vi "Dashboard Main.vi"() -> ()   [LabVIEW 2015]
uses:
  <vilib>/Utility/miscctls.llb/LVRowAndColumnTypeDef.ctl
  <vilib>/event_ctls.llb/eventvkey.ctl
  <vilib>/Rock Robotics/WPI/Dashboard/WPI_DashboardLogging Global.vi
  <vilib>/Rock Robotics/Network Tables/NT Read Numeric Array.vi
  <vilib>/Rock Robotics/Network Tables/NT Read Boolean.vi
  <vilib>/Utility/config.llb/Write Key (String).vi
  <vilib>/Utility/config.llb/Write Key (I32).vi
  <vilib>/Utility/config.llb/NI_LVConfig.lvlib
panel:
  in  "TCP":refnum<k5>
  in  "Rec Mode":enum32{"Stop", "Record", "Playback"}(radio)
  in  "Vision":u16(ring) items=["Camera Off", "USB Camera SW", "USB Camera HW", "IP Camera"]
  out "Camera IP":string
  out "Image Message":string="Timeout in Camera Communications"
  in  "Dashboard Tab":T1(tab)
  in  "Select Auto":string(combo)
  out "NT Connection":bool
  in  "Camera Settings":T2={"Frame Rate"=30, "Compression"=30, "Size"=1} {"Frame Rate" scale=1.0..30.0; "Size" items=["640x480", "320x240", "160x120"]}
  out "MotorChart R":cluster{"Numeric":dbl, "Numeric":dbl}(graph)
  out "MotorChart L":T3(graph)
  out "MotorSliders R":cluster{"MotorSlide1":dbl, "MotorSlide2":dbl} {"MotorSlide2" scale=-1.0..1.0 scale format="%#_2e"; "MotorSlide1" scale=-1.0..1.0 scale format="%#_2e"}
  out "MotorSliders L":T4 {"MotorSlide4 2" scale=0.0..14.0 scale format="%#_2e"; "MotorSlide2" scale=-1.0..1.0 scale format="%#_2e"; "MotorSlide1" scale=-1.0..1.0 scale format="%#_2e"}
  out "Gyro":dbl(knob) scale=0.0..360.0
  out "JS1 Z":dbl(slide) scale=-1.0..1.0 scale format="%#_2e"
  out "JS1 Graph":cluster{"X":dbl, "Y":dbl}[](graph)
  out "JS1 Buttons":T5
  out "JS2 Z":dbl(slide) scale=-1.0..1.0 scale format="%#_2e"
  out "JS2 Graph":cluster{"X":dbl, "Y":dbl}[](graph)
  out "JS2 Buttons":T5
  out "Mode":T6(ring)=enum."Auto Disabled"
  in  "DB Camera Config":bool
  out "fps":dbl format="%#.1g"
  out "Mbps":dbl format="%#.1g"
  out "Mbps LED":bool
  in  "DB/String 9":string
  in  "DB/String 8":string
  in  "DB/String 7":string
  in  "DB/String 6":string
  in  "DB/String 5":string
  in  "DB/String 4":string
  in  "DB/String 3":string
  in  "DB/String 2":string
  in  "DB/String 1":string
  in  "DB/String 0":string
  in  "DB/Slider 0":dbl(slide) scale=0.0..5.0
  in  "DB/Slider 1":dbl(slide) scale=0.0..5.0
  in  "DB/Slider 2":dbl(slide) scale=0.0..5.0
  in  "DB/Slider 3":dbl(slide) scale=0.0..5.0
  out "DB/LED 3":bool
  out "DB/LED 2":bool
  out "DB/LED 1":bool
  out "DB/LED 0":bool
  in  "DB/Button 3":bool
  in  "DB/Button 2":bool
  in  "DB/Button 1":bool
  in  "DB/Button 0":bool caption="New Name"
  in  "Position":enum16{"No Launch", "3"}(ring)
  in  "Defense":T7(ring)
  out "Air Pressure":dbl
  out "Ball In Catapult":bool
  out "Climbing Only":bool
  in  "Test Slider":dbl(slide) scale=0.0..100.0 scale format="%#_3g"
  in  "On/Off":bool caption="Solenoid"
  in  "Test Name":u16(ring) items=["Select the test to run..."]
  in  "Test Tree":string(tree)
  in  "Motor":cluster{"Value":dbl, "Enable":bool} {"Value" scale=-1.0..1.0 scale format="%#_3g"}
  out "Progress":T8 {"Test Progress" scale=0.0..100.0}
  in  "Rev/Fwd":cluster{"Forward":bool, "Reverse":bool}
  in  "Test Ring":u16(ring) items=["Monochrome", "Color"]
  out "Cmd Status":string
  in  "Execute Command":bool
  in  "Command Params":string[][](table)
  in  "Command Selection":i32(listbox)
  in  "CheckList":i32(listbox)
  out "Tree":string(tree)
  out "Camera Image":T9(plugin-control)
  out "Background":bool
  # "Left"
  # "Front"
  # "Right"
  # "Battery"
  # "Autonomus"
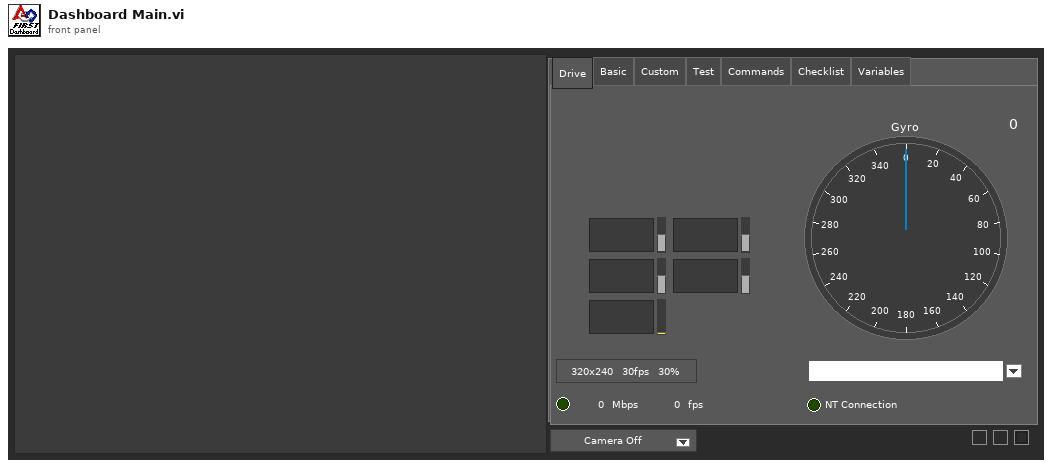
[diagram p1: front panel]
types:
  T1 = enum32{"Drive", "Basic", "Custom", "Test", "Commands", "Checklist", "Variables"}
  T2 = cluster{"Frame Rate":i32, "Compression":i32, "Size":u16}
  T3 = cluster{"Numeric":dbl, "Numeric":dbl, "Battery V":dbl}
  T4 = cluster{"MotorSlide1":dbl, "MotorSlide2":dbl, "MotorSlide4 2":dbl}
  T5 = cluster{bool, bool, bool, bool, bool, bool, bool, bool, bool, bool, bool, bool}
  T6 = enum8{"Tele-Op Disabled", "Tele-Op Enabled", "Auto Disabled", "Auto Enabled", "Test Disabled", "Test Enabled", "Disconnected", "No Code", "E-Stop"}
  T7 = enum16{"Rock Wall/Rough Terrain/Moat", "Ramp Parts", "Low Bar"}
  T8 = cluster{"Test Progress":u8, "Test Progress Text":string}
  T9 = typedef "IMAQ Image.ctl" = refnum<image>
  T10 = cluster{"IDs":cluster{"RPC field ID":u16, "Unique ID":u16}, "String":string}
  T11 = enum32{"Drive", "Basic", "Custom", "Test", "Checklist", "Variables"}
  T12 = typedef "Image Type" = u32
  T13 = cluster{"Camera Image":refnum<vi>, "Dashboard Tab":refnum<vi>, "Background":refnum<vi>, "Vision":refnum<vi>, "Rec Mode":refnum<vi>, "Test Slider":refnum<vi>, "On/Off ":refnum<vi>, "Test Ring":refnum<vi>, "Rev/Fwd":refnum<vi>, "Test Name":refnum<vi>, "Motor":refnum<vi>, "Progress":refnum<vi>, "CheckList":refnum<vi>, "Tree":refnum<vi>, "Test Tree":refnum<vi>, "Command Params":refnum<vi>, "Command Selection":refnum<vi>, "Execute Command":refnum<vi>, "Cmd Status":refnum<vi>}
  T14 = cluster{"Error Strings":string, "Disable Counts":cluster{u16, u16}, "Rail Faults":cluster{u16, u16, u16}, "Robot IP":string, "DB Mode":u8, "Event Info":cluster{"Name":string, "Type":u8, "Number":u16, "Replay":u8}, "Camera Addr":string}
  T15 = cluster{"Storage":cluster{"Disk Free":u64, "RAM Block":u32, "RAM free":u32}, "CPU Utilization":cluster{"CPU % ISR":sgl, "CPU % Time Crit":sgl, "CPU % Timed Str":sgl, "CPU % High":sgl, "CPU % Above":sgl, "CPU % Normal":sgl, "CPU % Low":sgl}, "CAN":cluster{"% Bus Utilization":sgl, "Bus Off Cnt":u32, "TX_FIFO Full Cnt":u32, "Receive Error Cnt":u8, "Transmit Error Cnt":u8}, "HID":cluster{"HID Outputs":u32, "Rumble Low":u16, "Rumble High":u16}[]}
  T16 = cluster{"Status bits":cluster{"Test Mode":bool, "Autonomous":bool, "Enabled":bool, "Code Start":bool, "Brownout":bool, "Reserved 2":bool, "Reserved 3":bool, "E-Stop":bool}, "Code Trace":cluster{"Disabled":bool, "TeleOp":bool, "Auto":bool, "Test":bool}, "Controller Type":enum16{"unknown", "cRIO", "roboRio"}, "Code?":enum16{"unknown", "noCode", "code"}, "Battery V":dbl}
  T17 = cluster{"Control Bits":cluster{"TestMode":bool, "Autonomous":bool, "Enabled":bool, "FMS Present":bool, bool, bool, bool, "E-Stop":bool}, "Team Station ":u8, "Countdown":sgl, "Joystick Values":cluster{"Axes":dbl[], "Buttons":bool[], "POVs":i16[]}[]}
  T18 = cluster{"Axes":dbl[], "Buttons":bool[], "POVs":i16[]}[]
  T19 = cluster{"Axes":dbl[], "Buttons":bool[], "POVs":i16[]}
  T20 = cluster{"Buttons[0]":bool, "Buttons[1]":bool, "Buttons[2]":bool, "Buttons[3]":bool, "Buttons[4]":bool, "Buttons[5]":bool, "Buttons[6]":bool, "Buttons[7]":bool, "Buttons[8]":bool, "Buttons[9]":bool, "Buttons[10]":bool, "Buttons[11]":bool}
  T21 = typedef "NI_LVConfig.lvlib/Config Data RefNum.ctl" = refnum<k1>
  T22 = cluster{"Operation":enum16{"Update", "Clear"}, "Color Box":u32}[]
  T23 = typedef "eventvkey.ctl" = enum16{"ASCII", "Enter", "Return", "Shift", "Ctrl", "Alt", "Cmd", "Opt", "Caps", "NumLock", "Clear", "Break", "Up", "Down", "Left", "Right", "Insert", "Delete", "Home", "End", "PageUp", "PageDown", "Escape", "Help", "Pause", "ScrollLock", "F1", "F2", "F3", "F4", "F5", "F6", "F7", "F8", "F9", "F10", "F11", "F12", "F13", "F14", "F15", "F16", "F17", "F18", "F19", "F20", "F21", "F22", "F23", "F24", "Play", "VolumeUp", "VolumeDown", "Mute", "Two Byte Char"}
  T24 = cluster{"Image Size":bool, "Image Type":bool, "Pixel Value":bool, "ROI Information":bool, "Zoom Factor":bool}
  T25 = enum8{"Enabled", "Disabled", "Disabled and Grayed Out"}
  T26 = cluster{"Operation":enum16{"Update", "Clear"}, "Color Box":u32}
  T27 = typedef "LVRowAndColumnTypeDef.ctl" = cluster{"Row":i32, "Column":i32}
  T28 = cluster{"Shift":bool, "Ctrl":bool, "Alt":bool, "Cmd":bool, "Opt":bool}
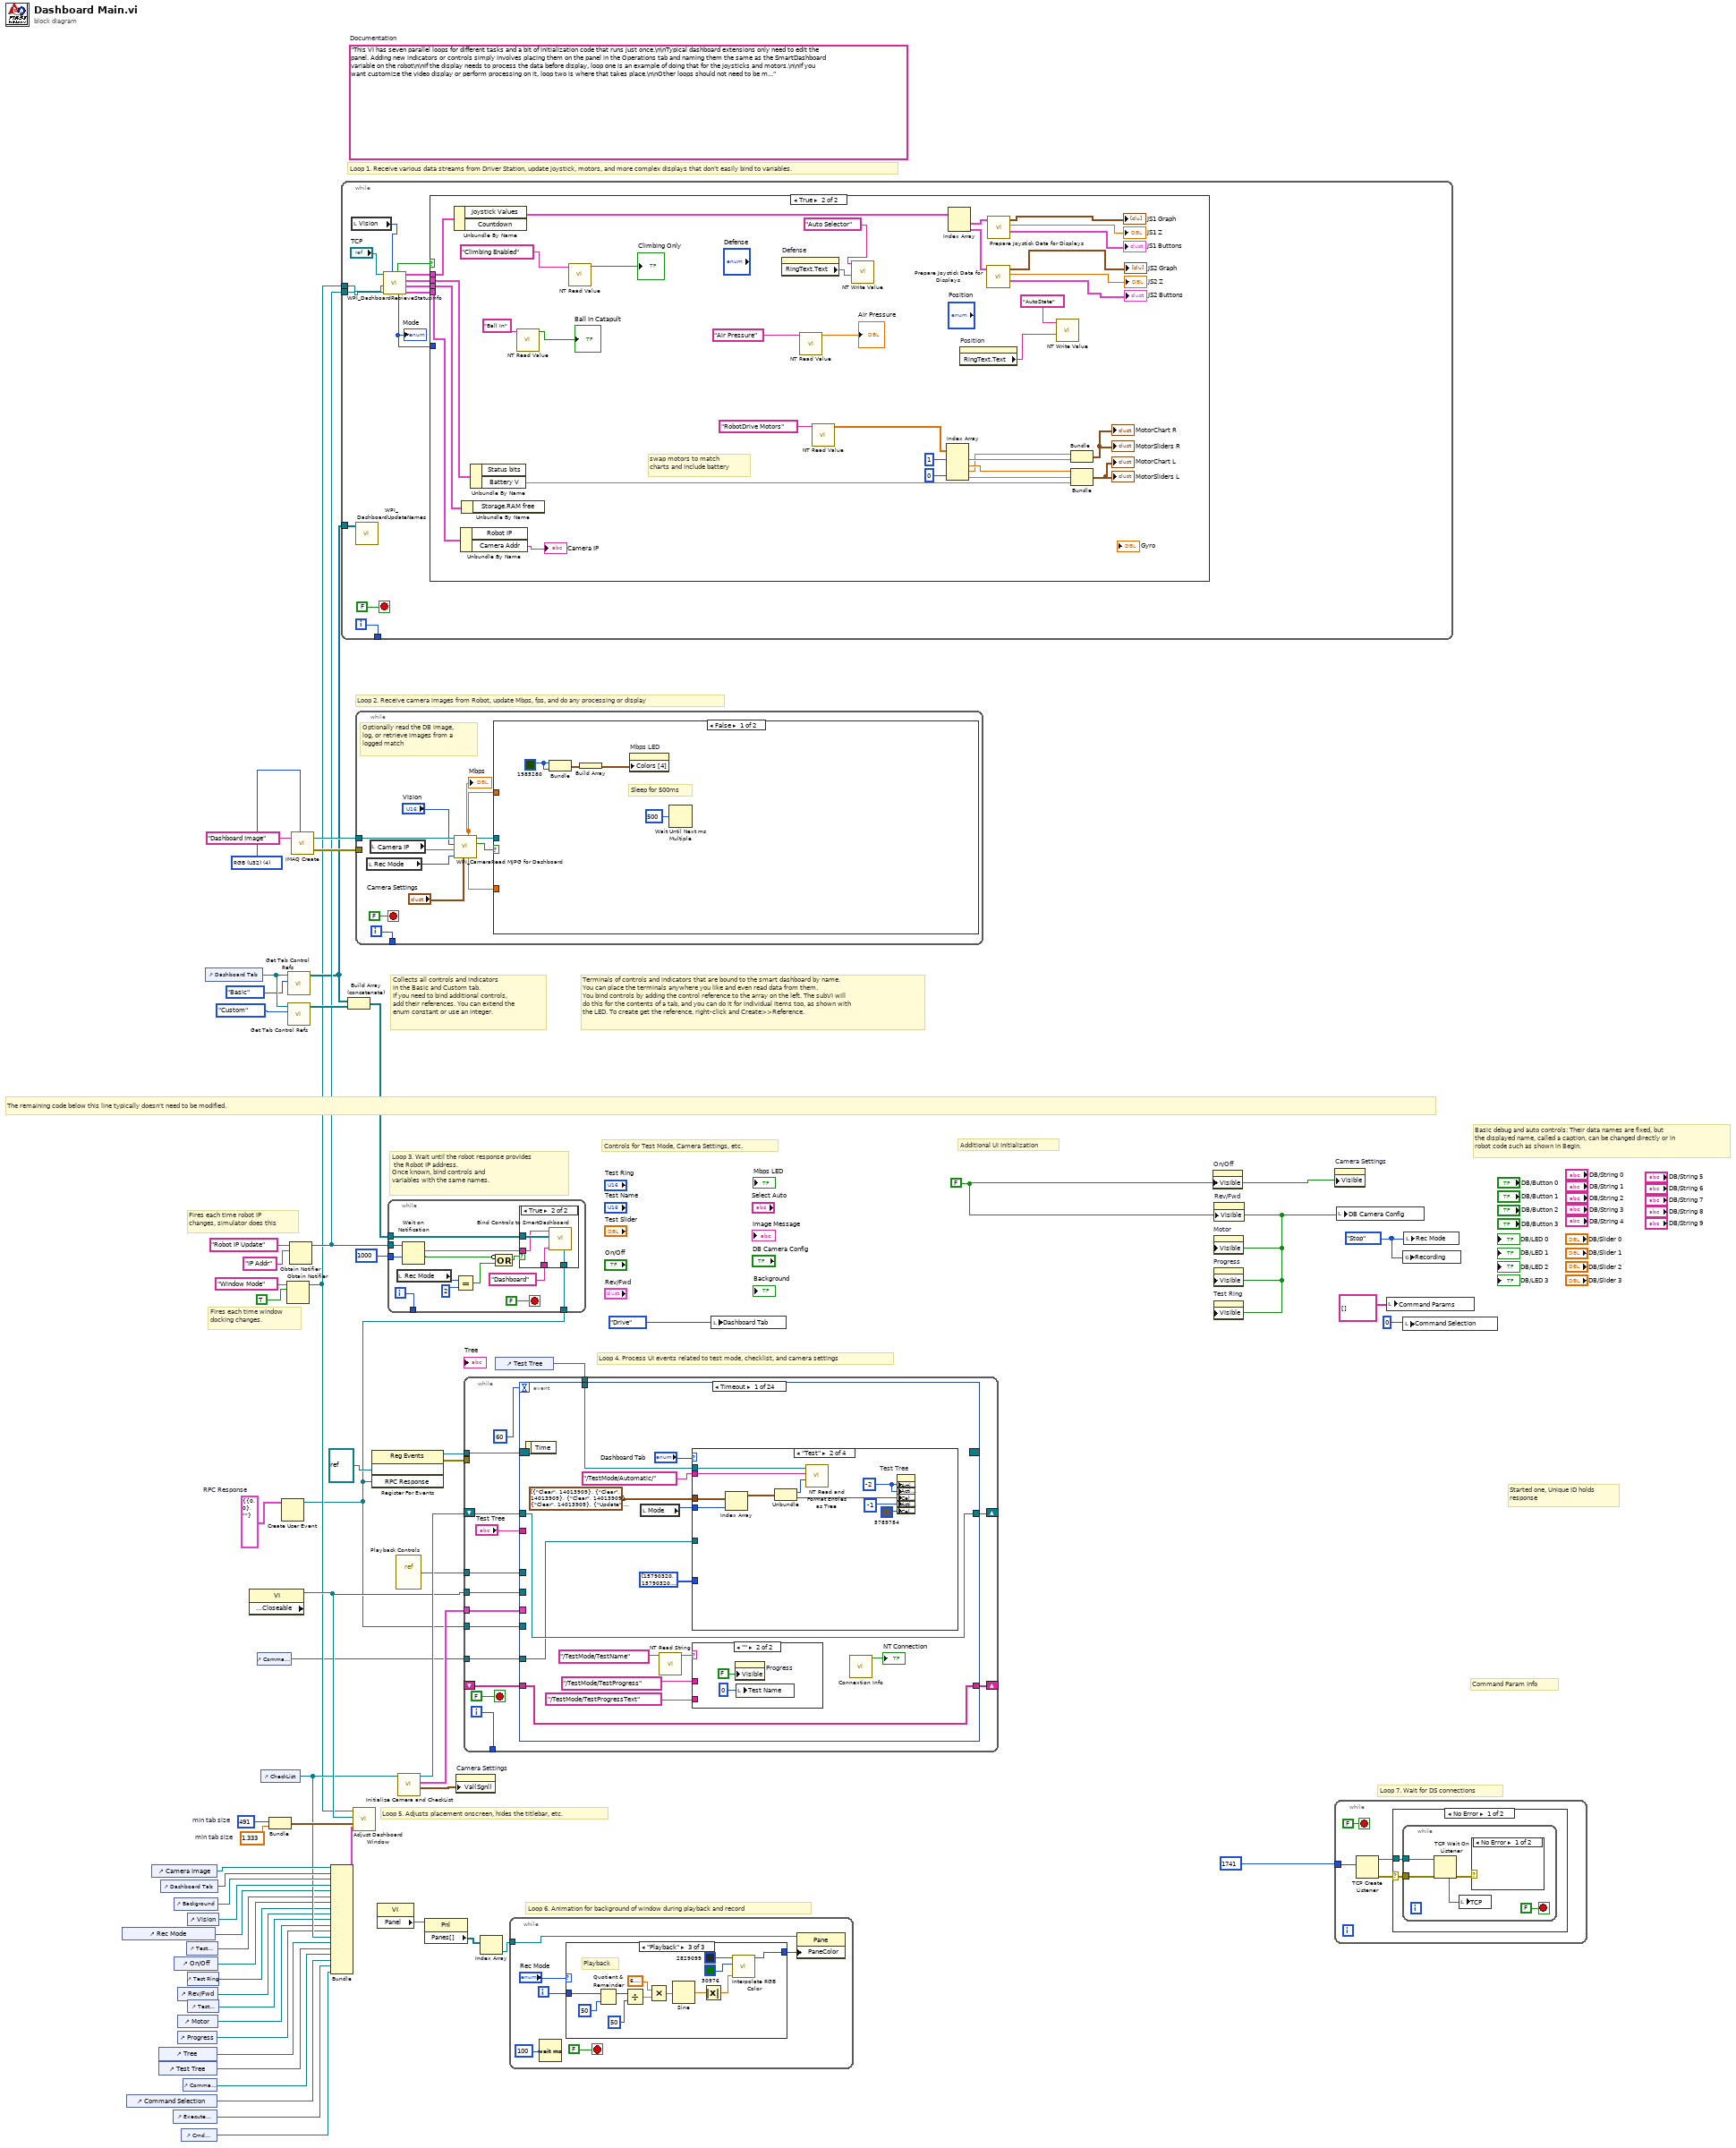
[diagram p0: block diagram]
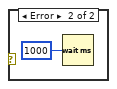
[diagram p2: hidden frame]
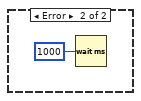
[diagram p3: hidden frame]
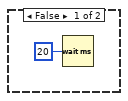
[diagram p4: hidden frame]
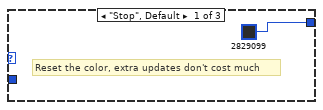
[diagram p5: hidden frame]
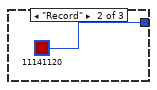
[diagram p6: hidden frame]
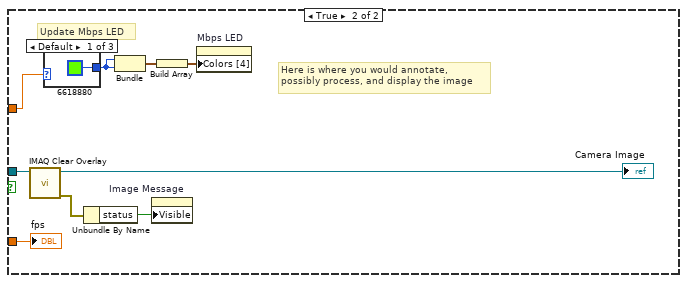
[diagram p8: hidden frame]
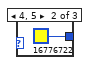
[diagram p9: hidden frame]
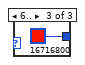
[diagram p10: hidden frame]
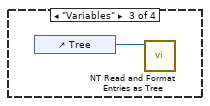
[diagram p12: hidden frame]
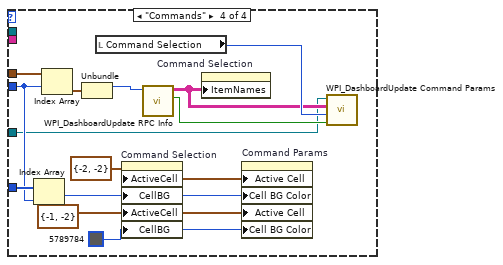
[diagram p13: hidden frame]
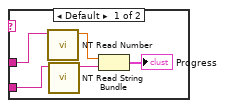
[diagram p14: hidden frame]
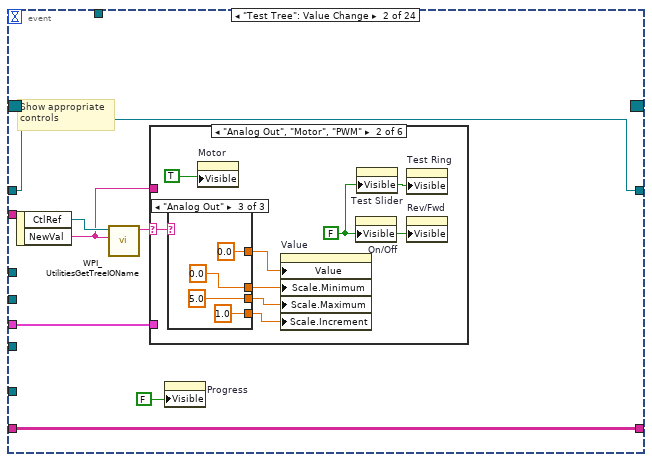
[diagram p15: hidden frame]
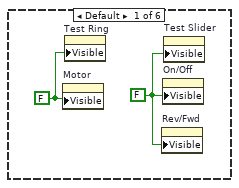
[diagram p16: hidden frame]
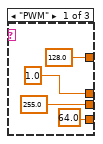
[diagram p17: hidden frame]
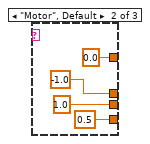
[diagram p18: hidden frame]
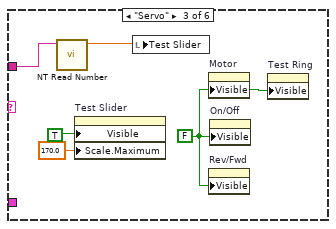
[diagram p19: hidden frame]
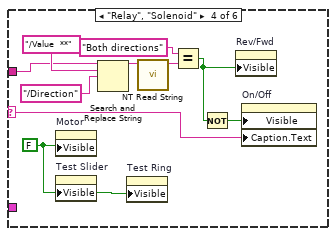
[diagram p20: hidden frame]
diagram:
  w7 = T10 {"IDs"={"RPC field ID"=0, "Unique ID"=0}, "String"=""}  # RPC Response
  w33 = 491  # min tab size
  w32 = 1.333  # min tab size
  w41 = enum32{"Stop", "Record", "Playback"}."Stop" ("Rec Mode")
  w15 = FALSE ("Visible")
  (unwired) "This VI has seven parallel loops for different tasks and a bit of initialization code that runs just once.\n\nTypical dashboard extensions only need to edit the panel. Adding new indicators or controls simply involves placing them on the panel in the Operations tab and naming them the same as the SmartDashboard variable on the robot\n\nIf the display needs to process the data before display, loop one is an example of doing that for the joysticks and motors.\n\nIf you want customize the video display or perform processing on it, loop two is where that takes place.\n\nOther loops should not need to be modified. They are pretty standard, and document the task they perform."  # Documentation
  w61 = T12 4 items=["Grayscale (U8)", "Grayscale (I16)", "Grayscale (SGL)", "Complex (CSG)", "RGB (U32)", "HSL (U32)", "RGB (U64)"] ("Image Type")
  # "Command Param Info"
  # "Started one, Unique ID holds\nresponse"
  # "Loop 7. Wait for DS connections"
  # "Basic debug and auto controls: Their data names are fixed, but\nthe displayed name, called a caption, can be changed directly or in\nrobot code such as shown in Begin."
  # "Controls for Test Mode, Camera Settings, etc."
  # "Additional UI Initialization"
  # "Loop 6. Animation for background of window during playback and record"
  # "Fires each time robot IP\nchanges, simulator does this"
  # "Fires each time window\ndocking changes."
  # "Collects all controls and indicators\nin the Basic and Custom tab.\nIf you need to bind additional controls,\nadd their references. You can extend the\nenum constant or use an integer."
  # "The remaining code below this line typically doesn't need to be modified."
  # "Loop 4. Process UI events related to test mode, checklist, and camera settings"
  # "Terminals of controls and indicators that are bound to the smart dashboard by name.\nYou can place the terminals anywhere you like and even read data from them.\nYou bind controls by adding the control reference to the array on the left. The subVI will\ndo this for the contents of a tab, and you can do it for individual items too, as shown with\nthe LED. To create get the reference, right-click and Create>>Reference."
  # "Loop 3. Wait until the robot response provides\n the Robot IP address.\nOnce known, bind controls and\nvariables with the same names."
  # "Loop 5. Adjusts placement onscreen, hides the titlebar, etc."
  # "Loop 1. Receive various data streams from Driver Station, update joystick, motors, and more complex displays that don't easily bind to variables."
  # "Loop 2. Receive camera images from Robot, update Mbps, fps, and do any processing or display"
  n1 = control-ref of="Rec Mode"() -> (w21:refnum<vi>)
  n2 = control-ref of="Command Selection"() -> (w6:refnum<vi>)
  n3 = control-ref of="Camera Image"() -> (w36:refnum<vi>)
  n4 = control-ref of="Tree"() -> (w25:refnum<vi>)
  n5 = control-ref of="Test Tree"() -> (w24:refnum<vi>)
  n6 = control-ref of="Dashboard Tab"() -> (w35:refnum<vi>)
  n7 = control-ref of="Execute Command"() -> (w8:refnum<vi>)
  n8 = control-ref of="Background"() -> (w30:refnum<vi>)
  n9 = control-ref of="On/Off"() -> (w19:refnum<vi>)
  n10 = control-ref of="Progress"() -> (w16:refnum<vi>)
  n11 = control-ref of="Rev/Fwd"() -> (w17:refnum<vi>)
  n12 = control-ref of="Motor"() -> (w22:refnum<vi>)
  n13 = control-ref of="Cmd Status"() -> (w2:refnum<vi>)
  n14 = control-ref of="Command Params"() -> (w9:refnum<vi>)
  n15 = control-ref of="Test Slider"() -> (w20:refnum<vi>)
  n16 = control-ref of="Vision"() -> (w34:refnum<vi>)
  n17 = control-ref of="Test Ring"() -> (w18:refnum<vi>)
  n18 = control-ref of="Test Name"() -> (w23:refnum<vi>)
  n19 = control-ref of="Dashboard Tab"() -> (w39:refnum<vi>)
  n20 = property class="VI" props=["Front Panel.Closeable"]() -> (reference out=w40:refnum<vi>)  [unwired: 2 in, 2 out]
  n21 = control-ref of="Command Params"() -> (w1:refnum<vi>)
  n22 = control-ref of="CheckList"() -> (w26:refnum<vi>)
  n23 = Bundle("min tab size"=w33, "min tab size"=w32) -> (w31:cluster{"min tab size":i32, "min tab size":dbl})  [unwired: 1 in]
  n24 = Create User Event(user event datatype=w7) -> (user event=w3:refnum<user-event>)  [unwired: 1 in, 1 out]
  n25 = Obtain Notifier(name (unnamed)="Window Mode", notification data type=TRUE) -> (notifier out=w12:refnum<notifier>)  [unwired: 2 in, 2 out]
  n26 = call <vilib>:"Get Tab Control Refs.vi"("Page Index"=T11."Basic" ("Dashboard Tab"), "TabControl in"=w39) -> ("ControlsOnPage"=w13:refnum<vi>[])  [unwired: 9 in]
  n27 = call <vilib>:"Get Tab Control Refs.vi"("Page Index"=T11."Custom" ("Dashboard Tab"), "TabControl in"=w39) -> ("ControlsOnPage"=w38:refnum<vi>[])  [unwired: 9 in]
  n28 = Obtain Notifier(name (unnamed)="Robot IP Update", notification data type="IP Addr" ("name (unnamed)")) -> (notifier out=w14:refnum<notifier>)  [unwired: 2 in, 2 out]
  n29 = call "IMAQ Create"("Image Name"="Dashboard Image", "Image Type"=w61) -> ("New Image"=w59:T9, "error out"=w58:errorcluster)  [unwired: 2 in, 1 out]
  n30 = Bundle("Camera Image"=w36, "Dashboard Tab"=w35, "Background"=w30, "Vision"=w34, "Rec Mode"=w21, "Test Slider"=w20, "On/Off"=w19, "Test Ring"=w18, "Rev/Fwd"=w17, "Test Name"=w23, "Motor"=w22, "Progress"=w16, "CheckList"=w26, "Tree"=w25, "Test Tree"=w24, "Command Params"=w9, "Command Selection"=w6, "Execute Command"=w8, "Cmd Status"=w2) -> (w27:T13)  [unwired: 1 in]
  n31 = while {
    tunnel: [w73] -> _
    tunnel: w14 -> [w67]
    tunnel: w13 -> [w66]
    tunnel: w12 -> [w62]
    i -> [w73]
    stop <- FALSE stop-if-true
    n32 = local read "Vision"() -> (w64:u16)
    n33 = call <vilib>:"WPI_DashboardUpdateNames.vi"("Controls on Tab"=w66) -> ()  [unwired: 11 in]
    n34 = call <vilib>:"WPI_DashboardRetrieveStatusInfo.vi"("Vision"=w64, "Binding Refnum"=w67, "Window Mode Notifier"=w62, "TCP Cnx"="TCP") -> ("Power and Errors"=w68:T14, "Robot Metrics"=w71:T15, "Status Info"=w72:T16, "Control Info"=w69:T17, "Robot Mode"=w65:T6, "Process?"=w70:bool)  [unwired: 2 in]
    "Mode" <- w65
    n35 = case shown="True" w70 {
      tunnel: w72 -> [_ w110]
      tunnel: w71 -> [_ w109]
      tunnel: w69 -> [_ w108]
      tunnel: w68 -> [_ w107]
      tunnel: w65 -> [_ _]
      frame False {
        n36 = Wait (ms)(milliseconds to wait=u32 20) -> ()  [unwired: 1 out]
      }
      frame True {
        # "swap motors to match\ncharts and include battery"
        n37 = Unbundle By Name(w108) -> ("Joystick Values"=w97:T18)  [unwired: 1 out]
        n38 = Unbundle By Name(w107) -> ("Camera Addr"=→"Camera IP":string)  [unwired: 1 out]
        n39 = Unbundle By Name(w109) -> ()  [unwired: 1 out]
        n40 = Unbundle By Name(w110) -> ("Battery V"=w98:dbl)  [unwired: 1 out]
        n41 = call-poly <vilib>:"NT Read Value.vi"("Name"="Ball In") -> ("Boolean"=→"Ball In Catapult":bool)  [unwired: 9 in, 1 out]
        n42 = call-poly <vilib>:"NT Read Value.vi"("Name"="Climbing Enabled") -> ("Boolean"=→"Climbing Only":bool)  [unwired: 9 in, 1 out]
        n43 = property on="Defense" class="Enum (strict)"() -> ("RingText.Text"=w78:string)  [unwired: 2 in, 2 out]
        n44 = call-poly <vilib>:"NT Read Value.vi"("Name"="Air Pressure") -> ("Numeric"=→"Air Pressure":dbl)  [unwired: 9 in, 1 out]
        n45 = call-poly <vilib>:"NT Read Value.vi"("Name"="RobotDrive Motors") -> ("Numeric Array"=w86:dbl[])  [unwired: 9 in, 1 out]
        n46 = call-poly <vilib>:"NT Write Value.vi"("String"=w78, "Name"="Auto Selector") -> ()  [unwired: 9 in, 1 out]
        n47 = Index Array(array=w86, index #1=1, index #4=0) -> (element #1=w102:dbl, element #2=w103:dbl, element #3=w101:dbl, element #4=w106:dbl)  [unwired: 2 in]
        n48 = Index Array(array=w97) -> (element #1=w96:T19, element #2=w91:T19)  [unwired: 2 in]
        n49 = property on="Position" class="Enum (strict)"() -> ("RingText.Text"=w77:string)  [unwired: 2 in, 2 out]
        n50 = call "Prepare Joystick Data for Displays.vi"("Joystick Values"=w91) -> ("Buttons"=→"JS2 Buttons":T20, "Z Axis"=→"JS2 Z":dbl, "Cartesian Data"=→"JS2 Graph":cluster{"X axis":dbl, "X axis":dbl}[])  [unwired: 8 in]
        n51 = call "Prepare Joystick Data for Displays.vi"("Joystick Values"=w96) -> ("Buttons"=→"JS1 Buttons":T20, "Z Axis"=→"JS1 Z":dbl, "Cartesian Data"=→"JS1 Graph":cluster{"X axis":dbl, "X axis":dbl}[])  [unwired: 8 in]
        n52 = call-poly <vilib>:"NT Write Value.vi"("String"=w77, "Name"="AutoState") -> ()  [unwired: 9 in, 1 out]
        n53 = Bundle("Numeric"=w101, "Numeric"=w102) -> (→"MotorChart R" →"MotorSliders R":cluster{"Numeric":dbl, "Numeric":dbl})  [unwired: 1 in]
        n54 = Bundle("Numeric"=w103, "Numeric"=w106, "Battery V"=w98) -> (→"MotorChart L" →"MotorSliders L":T3)  [unwired: 1 in]
      }
    }
  }
  n55 = Build Array (concatenate)(w13, w38) -> (w37:refnum<vi>[])
  n56 = call "Adjust Dashboard Window.vi"("Sizing Refnums"=w27, "Size Constraints"=w31, "VI"=w40, "WIn Mode"=w12) -> ()  [unwired: 8 in]
  n57 = while {
    tunnel: w59 -> [w119]
    tunnel: w58 -> [_]
    tunnel: [w120] -> _
    i -> [w120]
    stop <- FALSE stop-if-true
    # "Optionally read the DB image,\nlog, or retrieve images from a\nlogged match"
    n58 = local read "Rec Mode"() -> (w114:enum32{"Stop", "Record", "Playback"})
    n59 = local read "Camera IP"() -> (w112:string)
    n60 = call <vilib>:"WPI_CameraRead MJPG for Dashboard.vi"("Camera Settings"="Camera Settings", "Rec Mode"=w114, "Camera IP"=w112, "Camera Mode"="Vision", "Refnum in"=w119) -> ("Active"=w117:bool, "Refnum out"=w118:T9, "FPS"=w116:dbl, "Bandwidth (Mbps)"=w111:dbl)  [unwired: 3 in]
    "Mbps" <- w111
    n61 = case shown="False" w117 {
      tunnel: w118 -> [_ w129]
      tunnel: w111 -> [_ w128]
      tunnel: w116 -> [_ w126]
      frame False {
        w122 = u32 1985280 ("Color Box")
        # "Sleep for 500ms"
        n62 = Bundle("Color Box"=w122, "Color Box"=w122) -> (w124:cluster{"Color Box":u32, "Color Box":u32})  [unwired: 1 out]
        n63 = Build Array(w124) -> (w123:cluster{"Color Box":u32, "Color Box":u32}[])
        n64 = property on="Mbps LED" class="Bool (strict)"("Colors [4]"=w123) -> ()  [unwired: 2 in, 2 out]
        n65 = Wait Until Next ms Multiple(millisecond multiple=u32 500) -> ()  [unwired: 1 out]
      }
      frame True {
        # "Here is where you would annotate,\npossibly process, and display the image"
        # "Update Mbps LED"
        n66 = call "IMAQ Clear Overlay"("Image"=w129) -> ("error out"=w133:errorcluster, "Image Out"=→"Camera Image":T9)  [unwired: 2 in, 7 out]
        n67 = case shown="Default" w128 {
          tunnel: [u32 6618880 ("Color Box") u32 16776722 ("Color Box") u32 16716800 ("Color Box")] -> w130
          frame Default {
          }
          frame 4, 5 {
          }
          frame 6.. {
          }
        }
        n68 = Unbundle By Name(w133) -> ("status"=w134:bool)
        n69 = Bundle("Color Box"=w130, "Color Box"=w130) -> (w132:cluster{"Color Box":u32, "Color Box":u32})  [unwired: 1 out]
        n70 = property on="Image Message" class="Str"("Visible"=w134) -> ()  [unwired: 2 in, 2 out]
        n71 = Build Array(w132) -> (w131:cluster{"Color Box":u32, "Color Box":u32}[])
        n72 = property on="Mbps LED" class="Bool (strict)"("Colors [4]"=w131) -> ()  [unwired: 2 in, 2 out]
        "fps" <- w126
      }
    }
  }
  n73 = register-events(refnum<vi> refnum, w3) -> (reference out=w45:refnum<event-registration>, error out=w44:errorcluster)  [unwired: 2 in]
  n74 = property class="VI"() -> ("Panel"=w48:refnum<vi>)  [unwired: 2 in, 2 out]
  n75 = while {
    tunnel: w37 -> [w150]
    tunnel: w14 -> [w148]
    tunnel: [w146] -> _
    tunnel: u32 1000 ("milliseconds to wait") -> [w145]
    tunnel: w3 -> [w138]
    i -> [w146]
    stop <- FALSE stop-if-true
    n76 = local read "Rec Mode"() -> (w141:enum32{"Stop", "Record", "Playback"})
    n77 = Wait on Notification(notifier=w148, timeout in ms (-1)=w145) -> (notification=w147:string, timed out?=w143:bool)  [unwired: 2 in, 2 out]
    n78 = Equal?(x=w141, y=u16 2 ("Rec Mode")) -> (x = y?=w142:bool)
    n79 = Compound Arithmetic op=OR(invert w143, w142) -> (w144:bool)
    n80 = case shown="True" w144 {
      tunnel: w150 -> [_ w154]
      tunnel: w147 -> [_ w153]
      tunnel: "Dashboard" -> [_ w152]
      tunnel: w138 -> [_ w151]
      frame False {
      }
      frame True {
        n81 = call <vilib>:"Bind Controls to SmartDashboard.vi"("RPC ref"=w151, "Client Name"=w152, "Bound Control Refs"=w154, "Server IP Address"=w153) -> ()  [unwired: 8 in]
      }
    }
  }
  n82 = vi-ref "Playback Controls.vi"() -> (w46:refnum<vi>)
  n83 = call "Initialize Camera and CheckList.vi"("ListBox in"=w26) -> ("Cluster"=w52:cluster{"value":i32, "value":i32, "index":i32}, "Array"=w53:cluster{string[]}[], "File Refnum"=w51:T21)  [unwired: 8 in]
  n84 = property class="Pnl"(reference=w48) -> ("Panes[]"=w49:refnum<vi>[])  [unwired: 1 in, 2 out]
  n85 = property on="Camera Settings" class="Clust (strict)"("Val(Sgnl)"=w52) -> ()  [unwired: 2 in, 2 out]
  n86 = Index Array(array=w49) -> (element=w47:refnum<vi>)  [unwired: 1 in]
  n87 = control-ref of="Test Tree"() -> (w50:refnum<vi>)
  n88 = while {
    tunnel: w53 -> [w166]
    shift-right: [w165] -> _
    shift-left: w51 -> [w164]
    tunnel: [w163] -> _
    tunnel: w50 -> [w162]
    tunnel: w46 -> [w161]
    tunnel: w45 -> [w160]
    tunnel: w44 -> [_]
    tunnel: w40 -> [w159]
    tunnel: w3 -> [w158]
    tunnel: w1 -> [w157]
    shift-right: [w156] -> _
    shift-left: _ -> [w155]
    i -> [w163]
    stop <- FALSE stop-if-true
    n89 = event shown="[0] Timeout" {
      selector: w160 -> [_ _ _ _ _ _ _ _ _ _ _ _ _ _ _ _ _ _ _ _ _ _ _ _]
      dyn-events: [_ _ _ _ _ _ _ _ _ _ _ _ _ _ _ _ _ _ w475 _ _ _ _ _] -> _
      timeout: u32 60 ("milliseconds to wait") -> [_ _ _ _ _ _ _ _ _ _ _ _ _ _ _ _ _ _ _ _ _ _ _ _]
      tunnel: w162 -> [w179 _ _ _ _ _ _ _ _ _ _ _ _ _ _ _ _ _ _ _ _ _ _ _]
      tunnel: "Test Tree" -> [_ _ _ _ _ _ _ _ _ _ _ _ _ w438 w447 w450 w455 w464 _ _ _ _ _ _]
      tunnel: w166 -> [_ w217 _ _ _ _ _ _ _ _ _ w400 w431 _ _ _ _ _ _ _ _ _ _ _]
      tunnel: [w176 w216 w320 w326 w336 w340 w346 w358 w366 w372 w385 w399 w424 w437 w445 w449 w454 w463 w477 w493 w495 w503 w514 w519] -> w165
      tunnel: w164 -> [w176 w216 w320 w326 w336 w340 w346 w358 w366 w372 w385 w398 w424 w437 w445 w449 w454 w463 w477 w493 w495 w503 w514 w519]
      tunnel: w161 -> [_ _ _ _ _ _ _ _ _ _ _ _ _ _ _ _ _ _ w478 _ w498 _ _ _]
      tunnel: w159 -> [_ _ _ _ _ _ _ _ _ _ _ _ _ _ _ _ _ _ w473 _ _ _ _ _]
      tunnel: w158 -> [_ _ _ _ _ _ _ _ _ _ _ _ _ _ _ _ _ _ w469 _ _ _ _ _]
      tunnel: w157 -> [w171 _ _ _ _ _ w344 _ _ _ _ _ _ _ _ _ _ _ _ _ _ _ _ _]
      tunnel: [w170 w215 w319 w325 w335 w341 w342 w352 w363 w371 w384 w397 w423 w436 w444 w448 w453 w462 w468 w491 w494 w499 w507 w520] -> w156
      tunnel: w155 -> [w170 w215 w319 w325 w335 w341 w342 _ _ w371 w384 w397 w423 w436 w444 w448 w453 w462 w468 w491 w494 w499 w507 w520]
      event Timeout {
        n90 = event-data() -> ()  [unwired: 1 in, 1 out]
        n91 = local read "Mode"() -> (w173:T6)
        n92 = call <vilib>:"NT Read String.vi"("Name"="/TestMode/TestName") -> ("String"=w182:string)  [unwired: 9 in, 1 out]
        n93 = case shown="\"Test\"" "Dashboard Tab" {
          tunnel: w179 -> [_ w193 _ _]
          tunnel: "/TestMode/Automatic/" ("Name Pattern") -> [_ w192 _ _]
          tunnel: T22 [{"Operation"=enum."Clear", "Color Box"=14013909}, {"Operation"=enum."Clear", "Color Box"=14013909}, {"Operation"=enum."Clear", "Color Box"=14013909}, {"Operation"=enum."Clear", "Color Box"=14013909}, {"Operation"=enum."Update", "Color Box"=14013909}, {"Operation"=enum."Update", "Color Box"=16777215}, {"Operation"=enum."Clear", "Color Box"=14013909}, {"Operation"=enum."Clear", "Color Box"=14013909}, {"Operation"=enum."Clear", "Color Box"=14013909}] -> [_ w185 _ w202]
          tunnel: w173 -> [_ w184 _ w201]
          tunnel: u32[] [15790320, 15790320, 15790320, 15790320, 16777215, 16777215, 15790320, 15790320, 15790320] -> [_ _ _ w207]
          tunnel: w171 -> [_ _ _ w195]
          frame "Custom", Default {
          }
          frame "Test" {
            w191 = -2 ("Active Item:Row Number")
            n94 = Index Array(array=w185, index=w184) -> (element=w186:T26)
            n95 = Unbundle(w186) -> ("Operation"=w187:enum16{"Update", "Clear"}, "Color Box"=w188:u32)
            n96 = call <vilib>:"NT Read and Format Entries as Tree.vi"("Operation"=w187, "Name Pattern"=w192, "Tree Refnum"=w193) -> ()  [unwired: 7 in, 2 out]
            n97 = property on="Test Tree" class="Tree (strict)"("Active Item Row Number"=w191, "ActiveColNum"=w191, "CellBG"=w188, "Active Item Row Number"=-1 ("Active Item:Row Number"), "CellBG"=u32 5789784 ("Color Box")) -> ()  [unwired: 2 in, 2 out]
          }
          frame "Variables" {
            n98 = control-ref of="Tree"() -> (w194:refnum<vi>)
            n99 = call <vilib>:"NT Read and Format Entries as Tree.vi"("Tree Refnum"=w194) -> ()  [unwired: 9 in, 2 out]
          }
          frame "Commands" {
            w203 = u32 5789784 ("Color Box")
            w204 = T27 {"Row"=-1, "Column"=-2} ("Active Cell:Active Cell")
            w206 = T27 {"Row"=-2, "Column"=-2} ("Active Cell:Active Cell")
            n100 = Index Array(array=w207, index=w201) -> (element=w205:u32)
            n101 = Index Array(array=w202, index=w201) -> (element=w200:T26)
            n102 = Unbundle(w200) -> ("Operation"=w199:enum16{"Update", "Clear"})  [unwired: 1 out]
            n103 = local read "Command Selection"() -> (w198:i32)
            n104 = property on="Command Selection" class="MCListbox (strict)"("ActiveCell"=w206, "CellBG"=w205, "ActiveCell"=w204, "CellBG"=w203) -> ()  [unwired: 2 in, 2 out]
            n105 = call <vilib>:"WPI_DashboardUpdate RPC Info.vi"("Operation"=w199) -> ("update"=w197:bool, "commands"=w196:string[][])  [unwired: 9 in]
            n106 = property on="Command Selection" class="MCListbox (strict)"("ItemNames"=w196) -> ()  [unwired: 2 in, 2 out]
            n107 = property on="Command Params" class="Tbl (strict)"("Active Cell"=w206, "Cell BG Color"=w205, "Active Cell"=w204, "Cell BG Color"=w203) -> ()  [unwired: 2 in, 2 out]
            n108 = call <vilib>:"WPI_DashboardUpdate Command Params.vi"("Update"=w197, "NewVal"=w198, "Commands"=w196, "Param Tbl"=w195) -> ()  [unwired: 7 in, 1 out]
          }
        }
        n109 = case shown="\"\"" w182 {
          tunnel: "/TestMode/TestProgress" ("Name") -> [w209 _]
          tunnel: "/TestMode/TestProgressText" ("Name") -> [w208 _]
          frame Default {
            n110 = call <vilib>:"NT Read Number.vi"("Name"=w209) -> ("Numeric"=w210:dbl)  [unwired: 9 in, 1 out]
            n111 = call <vilib>:"NT Read String.vi"("Name"=w208) -> ("String"=w211:string)  [unwired: 9 in, 1 out]
            n112 = Bundle("Numeric"=w210, "String"=w211) -> (→"Progress":cluster{"Numeric":dbl, "String":string})  [unwired: 1 in]
          }
          frame "" {
            n113 = property on="Progress" class="Clust (strict)"("Visible"=FALSE) -> ()  [unwired: 2 in, 2 out]
            n114 = local write "Test Name"(u16 0) -> ()
          }
        }
        n115 = call <vilib>:"Connextion Info.vi"() -> ("Connected"=→"NT Connection":bool)  [unwired: 10 in, 1 out]
      }
      event "Test Tree": Value Change {
        # "Show appropriate\ncontrols"
        n116 = event-data() -> ("CtlRef"=w220:refnum<vi>, "NewVal"=w218:string)  [unwired: 1 in]
        n117 = call <vilib>:"WPI_UtilitiesGetTreeIOName.vi"("NewVal"=w218, "TreeControl in"=w220) -> ("I/O Name"=w221:string)  [unwired: 9 in]
        n118 = case shown="\"Analog Out\", \"Motor\", \"PWM\"" w221 {
          selector: w221 -> [_ w228 _ w250 w259 _]
          tunnel: w218 -> [_ _ w247 w249 _ w266]
          tunnel: w217 -> [_ _ _ _ _ w265]
          frame Default {
            w223 = FALSE ("Visible")
            w222 = FALSE ("Visible")
            n119 = property on="Motor" class="Clust (strict)"("Visible"=w222) -> ()  [unwired: 2 in, 2 out]
            n120 = property on="Test Ring" class="Ring (strict)"("Visible"=w222) -> ()  [unwired: 2 in, 2 out]
            n121 = property on="Rev/Fwd" class="Clust (strict)"("Visible"=w223) -> ()  [unwired: 2 in, 2 out]
            n122 = property on="On/Off" class="Bool (strict)"("Visible"=w223) -> ()  [unwired: 2 in, 2 out]
            n123 = property on="Test Slider" class="Slide (strict)"("Visible"=w223) -> ()  [unwired: 2 in, 2 out]
          }
          frame "Analog Out", "Motor", "PWM" {
            w229 = FALSE ("Visible")
            n124 = case shown="\"Analog Out\"" w228 {
              tunnel: [1.0 ("Value") -1.0 ("Value") 0.0 ("Value")] -> w227
              tunnel: [255.0 ("Value") 1.0 ("Value") 5.0 ("Value")] -> w226
              tunnel: [128.0 ("Value") 0.0 ("Value") 0.0 ("Value")] -> w225
              tunnel: [64.0 ("Value") 0.5 ("Value") 1.0 ("Value")] -> w224
              frame "PWM" {
              }
              frame "Motor", Default {
              }
              frame "Analog Out" {
              }
            }
            n125 = property on="Motor" class="Clust (strict)"("Visible"=TRUE) -> ()  [unwired: 2 in, 2 out]
            n126 = property on="Value" class="Slide (strict)"("Value"=w225, "Scale.Minimum"=w227, "Scale.Maximum"=w226, "Scale.Increment"=w224) -> ()  [unwired: 2 in, 2 out]
            n127 = property on="On/Off" class="Bool (strict)"("Visible"=w229) -> ()  [unwired: 2 in, 2 out]
            n128 = property on="Test Slider" class="Slide (strict)"("Visible"=w229) -> ()  [unwired: 2 in, 2 out]
            n129 = property on="Test Ring" class="Ring (strict)"("Visible"=w229) -> ()  [unwired: 2 in, 2 out]
            n130 = property on="Rev/Fwd" class="Clust (strict)"("Visible"=w229) -> ()  [unwired: 2 in, 2 out]
          }
          frame "Servo" {
            w245 = FALSE ("Visible")
            n131 = call <vilib>:"NT Read Number.vi"("Name"=w247) -> ("Numeric"=w246:dbl)  [unwired: 9 in, 1 out]
            n132 = property on="Test Slider" class="Slide (strict)"("Visible"=TRUE, "Scale.Maximum"=170.0 ("Scale.Range:Maximum")) -> ()  [unwired: 2 in, 2 out]
            n133 = local write "Test Slider"(w246) -> ()
            n134 = property on="Motor" class="Clust (strict)"("Visible"=w245) -> ()  [unwired: 2 in, 2 out]
            n135 = property on="Rev/Fwd" class="Clust (strict)"("Visible"=w245) -> ()  [unwired: 2 in, 2 out]
            n136 = property on="On/Off" class="Bool (strict)"("Visible"=w245) -> ()  [unwired: 2 in, 2 out]
            n137 = property on="Test Ring" class="Ring (strict)"("Visible"=w245) -> ()  [unwired: 2 in, 2 out]
          }
          frame "Relay", "Solenoid" {
            w248 = FALSE ("Visible")
            n138 = property on="Motor" class="Clust (strict)"("Visible"=w248) -> ()  [unwired: 2 in, 2 out]
            n139 = property on="Test Slider" class="Slide (strict)"("Visible"=w248) -> ()  [unwired: 2 in, 2 out]
            n140 = Search and Replace String(input string=w249, search string="/Value  **", replace string="/Direction") -> (result string=w255:string)  [unwired: 5 in, 3 out]
            n141 = property on="Test Ring" class="Ring (strict)"("Visible"=w248) -> ()  [unwired: 2 in, 2 out]
            n142 = call <vilib>:"NT Read String.vi"("Name"=w255) -> ("String"=w253:string)  [unwired: 9 in, 1 out]
            n143 = Equal?(x="Both directions", y=w253) -> (x = y?=w251:bool)
            n144 = Not(x=w251) -> (.not. x?=w252:bool)
            n145 = property on="Rev/Fwd" class="Clust (strict)"("Visible"=w251) -> ()  [unwired: 2 in, 2 out]
            n146 = property on="On/Off" class="Bool (strict)"("Visible"=w252, "Caption.Text"=w250) -> ()  [unwired: 2 in, 2 out]
          }
          frame "Compressor", "Digital Out" {
            w258 = FALSE ("Visible")
            # "Get direction and finish"
            n147 = property on="Motor" class="Clust (strict)"("Visible"=w258) -> ()  [unwired: 2 in, 2 out]
            n148 = property on="Test Slider" class="Slide (strict)"("Visible"=w258) -> ()  [unwired: 2 in, 2 out]
            n149 = property on="Test Ring" class="Ring (strict)"("Visible"=w258) -> ()  [unwired: 2 in, 2 out]
            n150 = property on="On/Off" class="Bool (strict)"("Visible"=TRUE, "Caption.Text"=w259) -> ()  [unwired: 2 in, 2 out]
            n151 = property on="Rev/Fwd" class="Clust (strict)"("Visible"=FALSE) -> ()  [unwired: 2 in, 2 out]
          }
          frame "Camera" {
            n152 = call <vilib>:"Get Last Path Segment.vi"("String in"=w266) -> ("String out"=w267:string)  [unwired: 10 in]
            n153 = property on="On/Off" class="Bool (strict)"("Visible"=FALSE) -> ()  [unwired: 2 in, 2 out]
            n154 = property on="Motor" class="Clust (strict)"("Visible"=FALSE) -> ()  [unwired: 2 in, 2 out]
            n155 = property on="Rev/Fwd" class="Clust (strict)"("Visible"=FALSE) -> ()  [unwired: 2 in, 2 out]
            n156 = case shown="\"White Balance  **\"" w267 {
              tunnel: w266 -> [w273 w282 w291 w300 w309 _ w315]
              tunnel: w265 -> [w271 w279 w288 w297 w306 _ _]
              frame "Size  **" {
                n157 = Index Array(array=w271) -> (element=w270:cluster{string[]})  [unwired: 1 in]
                n158 = call <vilib>:"NT Read String.vi"("Name"=w273) -> ("String"=w272:string)  [unwired: 9 in, 1 out]
                n159 = Unbundle(w270) -> (w268:string[])
                n160 = Match First String(2:w268, 3:w272) -> (0:w269:i32)  [unwired: 1 out]
                n161 = property on="Test Ring" class="Ring (strict)"("Value"=w269, "Strings []"=w268) -> ()  [unwired: 2 in, 2 out]
                n162 = property on="Test Ring" class="Ring (strict)"("Visible"=TRUE) -> ()  [unwired: 2 in, 2 out]
                n163 = property on="Test Slider" class="Slide (strict)"("Visible"=FALSE) -> ()  [unwired: 2 in, 2 out]
              }
              frame "White Balance  **" {
                n164 = Index Array(array=w279, index=1) -> (element=w280:cluster{string[]})
                n165 = call <vilib>:"NT Read String.vi"("Name"=w282) -> ("String"=w281:string)  [unwired: 9 in, 1 out]
                n166 = Unbundle(w280) -> (w277:string[])
                n167 = Match First String(2:w277, 3:w281) -> (0:w276:i32)  [unwired: 1 out]
                n168 = property on="Test Ring" class="Ring (strict)"("Value"=w276, "Strings []"=w277) -> ()  [unwired: 2 in, 2 out]
                n169 = property on="Test Ring" class="Ring (strict)"("Visible"=TRUE) -> ()  [unwired: 2 in, 2 out]
                n170 = property on="Test Slider" class="Slide (strict)"("Visible"=FALSE) -> ()  [unwired: 2 in, 2 out]
              }
              frame "Exposure  **" {
                n171 = Index Array(array=w288, index=2) -> (element=w289:cluster{string[]})
                n172 = call <vilib>:"NT Read String.vi"("Name"=w291) -> ("String"=w290:string)  [unwired: 9 in, 1 out]
                n173 = Unbundle(w289) -> (w285:string[])
                n174 = Match First String(2:w285, 3:w290) -> (0:w286:i32)  [unwired: 1 out]
                n175 = property on="Test Ring" class="Ring (strict)"("Value"=w286, "Strings []"=w285) -> ()  [unwired: 2 in, 2 out]
                n176 = property on="Test Ring" class="Ring (strict)"("Visible"=TRUE) -> ()  [unwired: 2 in, 2 out]
                n177 = property on="Test Slider" class="Slide (strict)"("Visible"=FALSE) -> ()  [unwired: 2 in, 2 out]
              }
              frame "Exposure Priority  **" {
                n178 = Index Array(array=w297, index=3) -> (element=w298:cluster{string[]})
                n179 = call <vilib>:"NT Read String.vi"("Name"=w300) -> ("String"=w299:string)  [unwired: 9 in, 1 out]
                n180 = Unbundle(w298) -> (w294:string[])
                n181 = Match First String(2:w294, 3:w299) -> (0:w295:i32)  [unwired: 1 out]
                n182 = property on="Test Ring" class="Ring (strict)"("Value"=w295, "Strings []"=w294) -> ()  [unwired: 2 in, 2 out]
                n183 = property on="Test Ring" class="Ring (strict)"("Visible"=TRUE) -> ()  [unwired: 2 in, 2 out]
                n184 = property on="Test Slider" class="Slide (strict)"("Visible"=FALSE) -> ()  [unwired: 2 in, 2 out]
              }
              frame "Color Enable  **" {
                n185 = Index Array(array=w306, index=4) -> (element=w307:cluster{string[]})
                n186 = call <vilib>:"NT Read String.vi"("Name"=w309) -> ("String"=w308:string)  [unwired: 9 in, 1 out]
                n187 = Unbundle(w307) -> (w303:string[])
                n188 = Match First String(2:w303, 3:w308) -> (0:w304:i32)  [unwired: 1 out]
                n189 = property on="Test Ring" class="Ring (strict)"("Value"=w304, "Strings []"=w303) -> ()  [unwired: 2 in, 2 out]
                n190 = property on="Test Ring" class="Ring (strict)"("Visible"=TRUE) -> ()  [unwired: 2 in, 2 out]
                n191 = property on="Test Slider" class="Slide (strict)"("Visible"=FALSE) -> ()  [unwired: 2 in, 2 out]
              }
              frame Default {
                n192 = property on="Test Ring" class="Ring (strict)"("Visible"=FALSE) -> ()  [unwired: 2 in, 2 out]
                n193 = property on="Test Slider" class="Slide (strict)"("Visible"=FALSE) -> ()  [unwired: 2 in, 2 out]
              }
              frame "Brightness  **", "Color Level  **", "Compression  **", "FPS  **", "Sharpness  **" {
                n194 = call <vilib>:"NT Read Number.vi"("Name"=w315) -> ("Numeric"=w314:dbl)  [unwired: 9 in, 1 out]
                n195 = local write "Test Slider"(w314) -> ()
                n196 = property on="Test Slider" class="Slide (strict)"("Visible"=TRUE, "Scale.Maximum"=100.0 ("Scale.Range:Maximum")) -> ()  [unwired: 2 in, 2 out]
                n197 = property on="Test Ring" class="Ring (strict)"("Visible"=FALSE) -> ()  [unwired: 2 in, 2 out]
              }
            }
          }
        }
        n198 = property on="Progress" class="Clust (strict)"("Visible"=FALSE) -> ()  [unwired: 2 in, 2 out]
      }
      event "Test Name": Mouse Enter {
        # "Populate the ring with the list of tests"
        n199 = event-data() -> ()  [unwired: 1 in, 1 out]
        n200 = call <vilib>:"NT Read String Array.vi"("Name"="/TestMode/TestList") -> ("String Array"=w324:string[])  [unwired: 9 in, 1 out]
        n201 = Build Array (concatenate)("Select the test to run...", w324) -> (w323:string[])
        n202 = property on="Test Name" class="Ring (strict)"("Strings []"=w323) -> ()  [unwired: 2 in, 2 out]
      }
      event "Test Name": Value Change {
        w327 = FALSE ("Visible")
        # "Tell the robot the test name to run"
        n203 = event-data() -> ("NewVal"=w331:u16)  [unwired: 1 in]
        n204 = property on="Test Name" class="Ring (strict)"() -> ("Strings []"=w332:string[])  [unwired: 2 in, 2 out]
        n205 = local write "Progress"(T8 {"Test Progress"=0, "Test Progress Text"=""} ("Progress")) -> ()
        n206 = Index Array(array=w332, index=w331) -> (element=w330:string)
        n207 = call <vilib>:"NT Write String.vi"("String"=w330, "Name"="/TestMode/TestName") -> ()  [unwired: 9 in, 1 out]
        n208 = property on="Progress" class="Clust (strict)"("Visible"=TRUE) -> ()  [unwired: 2 in, 2 out]
        n209 = property on="Motor" class="Clust (strict)"("Visible"=w327) -> ()  [unwired: 2 in, 2 out]
        n210 = property on="Test Slider" class="Slide (strict)"("Visible"=w327) -> ()  [unwired: 2 in, 2 out]
        n211 = property on="On/Off" class="Bool (strict)"("Visible"=w327) -> ()  [unwired: 2 in, 2 out]
        n212 = property on="Rev/Fwd" class="Clust (strict)"("Visible"=w327) -> ()  [unwired: 2 in, 2 out]
        n213 = property on="Test Ring" class="Ring (strict)"("Visible"=w327) -> ()  [unwired: 2 in, 2 out]
      }
      event "Select Auto": Mouse Enter {
        # "Populate the combo box with the list of autonomous options"
        n214 = event-data() -> ()  [unwired: 1 in, 1 out]
        n215 = call <vilib>:"NT Read String Array.vi"("Name"="Auto List") -> ("String Array"=w334:string[])  [unwired: 9 in, 1 out]
        n216 = property on="Select Auto" class="CmbBox"("Strings[]"=w334) -> ()  [unwired: 2 in, 2 out]
      }
      event "Select Auto": Value Change {
        # "User modified the Auto Selection. Write to NT variable so robot knows."
        n217 = event-data() -> ("NewVal"=w338:string)  [unwired: 1 in]
        n218 = call <vilib>:"NT Write String.vi"("String"=w338, "Name"="Auto Selector") -> ()  [unwired: 9 in, 1 out]
      }
      event "Command Selection": Value Change {
        # "Get the params and show in table"
        n219 = event-data() -> ("NewVal"=w345:i32)  [unwired: 1 in]
        n220 = property on="Command Selection" class="MCListbox (strict)"() -> ("ItemNames"=w343:string[][])  [unwired: 2 in, 2 out]
        n221 = call <vilib>:"WPI_DashboardUpdate Command Params.vi"("NewVal"=w345, "Commands"=w343, "Param Tbl"=w344) -> ()  [unwired: 8 in, 1 out]
      }
      event "Execute Command": Value Change {
        # "Started one, Unique ID holds\nresponse"
        n222 = event-data() -> ()  [unwired: 1 in, 1 out]
        n223 = property on="Command Selection" class="MCListbox (strict)"() -> ("ItemNames"=w357:string[][])  [unwired: 2 in, 2 out]
        n224 = Index Array(array=w357, index (row)="Command Selection", index (col)=0) -> (element=w355:string)
        n225 = call <vilib>:"Invoke Commands.vi"("Command Params"="Command Params", "Function Name"=w355) -> ("Params"=w351:u8, "Started"=w350:bool)  [unwired: 7 in, 1 out]
        n226 = Array Subset(array="Command Params", length (row)=w351) -> (w352:string[][])  [unwired: 3 in]
        n227 = Select(t="Executing" ("Cmd Status"), s=w350, f="" ("Cmd Status")) -> (s? t:f=→"Cmd Status":string)
      }
      event "Command Selection": Double Click {
        n228 = event-data() -> ("Row"=w367:i32)  [unwired: 1 in]
        n229 = property on="Command Selection" class="MCListbox (strict)"() -> ("ItemNames"=w370:string[][])  [unwired: 2 in, 2 out]
        n230 = local read "Command Params"() -> (w365:string[][])
        n231 = Index Array(array=w370, index (row)=w367, index (col)=0) -> (element=w368:string)
        n232 = call <vilib>:"Invoke Commands.vi"("Command Params"=w365, "Function Name"=w368) -> ("Params"=w364:u8, "Started"=w359:bool)  [unwired: 7 in, 1 out]
        n233 = Array Subset(array=w365, length (row)=w364) -> (w363:string[][])  [unwired: 3 in]
        n234 = Select(t="Executing" ("Cmd Status"), s=w359, f="" ("Cmd Status")) -> (s? t:f=w360:string)
        n235 = local write "Cmd Status"(w360) -> ()
      }
      event "CheckList": Double Click {
        # "Shift clears all"
        # "Update symbols on the listbox"
        n236 = event-data() -> ("PlatMods.Shift"=w373:bool, "Row"=w375:i32)  [unwired: 1 in]
        n237 = case shown="True" w373 {
          tunnel: w375 -> [w379 _]
          tunnel: 1 -> [w378 _]
          frame False {
            n238 = property on="CheckList" class="LstBox (strict)"() -> ("Item Symbols"=w377:i32[])  [unwired: 2 in, 2 out]
            n239 = Replace Array Subset(array=w377, new element=w378, index=w379) -> (w376:i32[])
            n240 = property on="CheckList" class="LstBox (strict)"("Item Symbols"=w376) -> ()  [unwired: 2 in, 2 out]
          }
          frame True {
            w380 = 0 ("Top Row")
            n241 = property on="CheckList" class="LstBox (strict)"() -> ("Number of Rows"=w382:u32)  [unwired: 2 in, 2 out]
            n242 = Initialize Array(0, w382) -> (w381:i32[])
            n243 = property on="CheckList" class="LstBox (strict)"("Top Row"=w380, "Value"=w380, "Item Symbols"=w381) -> ()  [unwired: 2 in, 2 out]
          }
        }
      }
      event "CheckList": Key Down {
        # "Update symbols on the listbox\nLeft and right keys check and uncheck"
        n244 = event-data() -> ("VKey"=w387:T23)  [unwired: 1 in]
        n245 = case shown="\"Left\", \"Right\"" w387 {
          selector: w387 -> [w392 _]
          tunnel: eventvkey."Left" ("VKey") -> [w390 _]
          frame "Left", "Right" {
            n246 = Equal?(x=w390, y=w392) -> (x = y?=w391:bool)
            n247 = Select(t=0, s=w391, f=1) -> (s? t:f=w393:i32)
            n248 = property on="CheckList" class="LstBox (strict)"() -> ("Item Symbols"=w396:i32[])  [unwired: 2 in, 2 out]
            n249 = Replace Array Subset(array=w396, new element=w393, index="CheckList") -> (w395:i32[])
            n250 = property on="CheckList" class="LstBox (strict)"("Item Symbols"=w395) -> ()  [unwired: 2 in, 2 out]
          }
          frame Default {
          }
        }
      }
      event "DB Camera Config": Value Change {
        # "Show or hide the cluster of controls, store in ini file"
        n251 = event-data() -> ("NewVal"=w401:bool)  [unwired: 1 in]
        n252 = case shown="False" w401 {
          tunnel: w400 -> [w410 _]
          tunnel: [w403 w421] -> w399
          tunnel: w398 -> [w402 w421]
          frame False {
            w417 = "Camera"
            w420 = FALSE ("Visible")
            n253 = local read "Camera Settings"() -> (w409:T2)
            n254 = Index Array(array=w410) -> (element=w413:cluster{string[]})  [unwired: 1 in]
            n255 = Unbundle(w409) -> ("Frame Rate"=w408:i32, "Compression"=w407:i32, "Size"=w411:u16)
            n256 = Unbundle(w413) -> (w412:string[])
            n257 = Index Array(array=w412, index=w411) -> (element=w406:string)
            n258 = call-poly <vilib>:"Write Key.vi"("section"=w417, "value"=w406, "key"="Size", "refnum"=w402) -> ("refnum out"=w419:T21)  [unwired: 2 in, 5 out]
            n259 = call-poly <vilib>:"Write Key.vi"("section"=w417, "value"=w408, "key"="FrameRate", "refnum"=w419) -> ("refnum out"=w418:T21)  [unwired: 1 in, 6 out]
            n260 = property on="Camera Settings" class="Clust (strict)"("Visible"=w420) -> ()  [unwired: 2 in, 2 out]
            n261 = local write "DB Camera Config"(w420) -> ()
            n262 = call-poly <vilib>:"Write Key.vi"("section"=w417, "value"=w407, "key"="Compression", "refnum"=w418) -> ("refnum out"=w404:T21)  [unwired: 1 in, 6 out]
            n263 = call <vilib>:"Close Config Data.vi"("refnum"=w404) -> ("file path"=w405:path)  [unwired: 2 in, 8 out]
            n264 = call <vilib>:"Open Config Data.vi"("configuration file path"=w405) -> ("refnum"=w403:T21)  [unwired: 8 in, 2 out]
          }
          frame True {
            n265 = property on="Camera Settings" class="Clust (strict)"("Visible"=TRUE) -> ()  [unwired: 2 in, 2 out]
          }
        }
      }
      event "Camera Settings": Value Change {
        # "Update summary string when any elements of DB camera change"
        n266 = event-data() -> ("NewVal"=w435:T2)  [unwired: 1 in]
        n267 = Index Array(array=w431) -> (element=w430:cluster{string[]})  [unwired: 1 in]
        n268 = Unbundle(w435) -> ("Frame Rate"=w426:i32, "Compression"=w425:i32, "Size"=w428:u16)
        n269 = Unbundle(w430) -> (w429:string[])
        n270 = Index Array(array=w429, index=w428) -> (element=w427:string)
        n271 = Format Into String(format string="%s   %dfps   %d%%", w427, w426, w425) -> (resulting string=w432:string)  [unwired: 2 in, 1 out]
        n272 = Build Array(w432) -> (w433:string[])
        n273 = property on="DB Camera Config" class="Bool (strict)"("Strings [4]"=w433) -> ()  [unwired: 2 in, 2 out]
      }
      event "Motor.Enable": Value Change {
        # "When the test mode otor enable helper is set, update that\ntree row item's value"
        n274 = event-data() -> ("NewVal"=w442:bool)  [unwired: 1 in]
        n275 = Unbundle("Motor") -> ("Value"=w441:dbl)  [unwired: 1 out]
        n276 = Select(t=w441, s=w442, f=0.0) -> (s? t:f=w439:dbl)
        n277 = call <vilib>:"NT Write Number.vi"("Numeric"=w439, "Name"=w438) -> ()  [unwired: 9 in, 1 out]
      }
      event "Test Slider": Value Change {
        # "When the test mode slider helper is set, update that\ntree row item's value"
        n278 = event-data() -> ("NewVal"=w446:dbl)  [unwired: 1 in]
        n279 = call <vilib>:"NT Write Number.vi"("Numeric"=w446, "Name"=w447) -> ()  [unwired: 9 in, 1 out]
      }
      event "On/Off": Value Change {
        # "When the test mode on/off helper value is set, update that\ntree row item's value"
        n280 = event-data() -> ("NewVal"=w452:bool)  [unwired: 1 in]
        n281 = Boolean To (0,1)(Boolean=w452) -> (0, 1=w451:i16)
        n282 = call <vilib>:"NT Write Number.vi"("Numeric"=w451, "Name"=w450) -> ()  [unwired: 9 in, 1 out]
      }
      event "Rev/Fwd": Value Change {
        # "When the test mode helper value for relays is set, update that\ntree row item's value"
        n283 = event-data() -> ("NewVal.Forward"=w461:bool, "NewVal.Reverse"=w460:bool)  [unwired: 1 in]
        n284 = Boolean To (0,1)(Boolean=w461) -> (0, 1=w457:i16)
        n285 = Boolean To (0,1)(Boolean=w460) -> (0, 1=w459:i16)
        n286 = Negate(x=w459) -> (-x=w458:i16)
        n287 = Add(x=w457, y=w458) -> (x+y=w456:i16)
        n288 = call <vilib>:"NT Write Number.vi"("Numeric"=w456, "Name"=w455) -> ()  [unwired: 9 in, 1 out]
      }
      event "Test Ring": Value Change {
        # "When a test mode helper value is selected from the ring,\nset the tree item's variable to the string value"
        n289 = event-data() -> ("NewVal"=w466:u16)  [unwired: 1 in]
        n290 = property on="Test Ring" class="Ring (strict)"() -> ("Strings []"=w467:string[])  [unwired: 2 in, 2 out]
        n291 = Index Array(array=w467, index=w466) -> (element=w465:string)
        n292 = call <vilib>:"NT Write String.vi"("String"=w465, "Name"=w464) -> ()  [unwired: 9 in, 1 out]
      }
      event "Rec Mode": Value Change {
        # "Update globals for recording mode and path to read log from.\nClear when logging and let NetworkTables set path for vision to\nuse."
        n293 = event-data() -> ("NewVal"=w479:enum32{"Stop", "Record", "Playback"})  [unwired: 1 in]
        n294 = global write "WPI_DashboardLogging Global.vi" "Logging Filename"(path "") -> ()
        n295 = global write "WPI_DashboardLogging Global.vi" "Recording"(w479) -> ()
        n296 = case shown="\"Playback\"" w479 {
          tunnel: w478 -> [_ w481 w490]
          tunnel: [_ _ w489] -> w475
          tunnel: [_ _ w488] -> _
          tunnel: w473 -> [_ _ w486]
          tunnel: cluster{i32, i32} {-250, 170} -> [_ _ w485]
          tunnel: [_ _ T24 {"Image Size"=TRUE, "Image Type"=TRUE, "Pixel Value"=TRUE, "ROI Information"=TRUE, "Zoom Factor"=FALSE} ("Image Information Shown:All Elements")] -> w471
          tunnel: [_ _ TRUE ("Zoom Factor")] -> w470
          tunnel: w469 -> [_ _ w482]
          frame Default {
          }
          frame "Stop", "Record" {
            # "Place Window too"
            n297 = invoke class="VI" method="FP.Close"(reference=w481) -> (reference out=w480:refnum<vi>)  [unwired: 2 in, 2 out]
            n298 = invoke class="VI" method="Abort VI"(reference=w480) -> ()  [unwired: 2 in, 3 out]
          }
          frame "Playback" {
            n299 = call "Open Playback Panel.vi"("Offset"=w485, "DB VI Ref"=w486, "Playback in"=w490) -> ("Playback out"=w487:refnum<vi>)  [unwired: 8 in]
            n300 = register-events(w487, w482) -> (reference out=w489:refnum<event-registration>, error out=w488:errorcluster)  [unwired: 2 in]
          }
        }
        n301 = property on="Camera Image" class="ImageControl"("Image Information Shown"=w471, "Image Information Visible"=w470) -> ()  [unwired: 2 in, 2 out]
        n302 = call <vilib>:"WPI_DashboardNT Log FieldName Cache.vi"("Operation"=enum16{"Lookup/Add", "Index", "Clear"}."Clear") -> ()  [unwired: 8 in, 3 out]
      }
      event Panel Close {
        w492 = enum32{"Stop", "Record", "Playback"}."Stop" ("Rec Mode")
        # "Playback window has been closed, abort"
        n303 = event-data() -> ()  [unwired: 1 in, 4 out]
        n304 = local write "Rec Mode"(w492) -> ()
        n305 = global write "WPI_DashboardLogging Global.vi" "Recording"(w492) -> ()
      }
      event Panel Close {
        # "Abort playback window and ourself"
        n306 = event-data() -> ()  [unwired: 1 in, 4 out]
        n307 = invoke class="VI" method="FP.Close"(reference=w498) -> (reference out=w497:refnum<vi>)  [unwired: 2 in, 2 out]
        n308 = invoke class="VI" method="Abort VI"(reference=w497) -> (error out=w496:errorcluster)  [unwired: 2 in, 2 out]
        n309 = invoke class="VI" method="Abort VI"(error in=w496) -> ()  [unwired: 2 in, 3 out]
      }
      event User Event {
        n310 = event-data() -> ("IDs"=w506:cluster{"RPC field ID":u16, "Unique ID":u16}, "String"=w505:string)  [unwired: 1 in]
        n311 = Bundle("IDs"=w506, "String"=w505) -> (w504:T10)  [unwired: 1 in]
        n312 = call <vilib>:"Retrieve RPC Response.vi"("RPC Response"=w504) -> ("Output"=w501:string[][])  [unwired: 10 in]
        n313 = Build Array (concatenate)(w499, w501) -> (w500:string[][])
        n314 = local write "Command Params"(w500) -> ()
        n315 = local write "Cmd Status"("" ("Cmd Status")) -> ()
      }
      event "Vision": Value Change {
        # "Enable/Disable Compression slider.\nHW USB is hard-coded into the camera"
        n316 = event-data() -> ("NewVal"=w513:u16)  [unwired: 1 in]
        n317 = Equal?(x=w513, y=u32 2 ("milliseconds to wait")) -> (x = y?=w511:bool)
        n318 = Select(t=T25."Disabled and Grayed Out" ("Disabled"), s=w511, f=T25."Enabled" ("Disabled")) -> (s? t:f=w508:T25)
        n319 = property on="Compression" class="Slide (strict)"("DisabledEnum"=w508) -> ()  [unwired: 2 in, 2 out]
      }
      event "Tree": Double Click {
        n320 = event-data() -> ("PlatMods"=w518:T28, "Tag"=w517:string)  [unwired: 1 in]
        n321 = Unbundle(w518) -> ("Shift"=w516:bool)  [unwired: 4 out]
        n322 = Not(x=w516) -> (.not. x?=w515:bool)
        n323 = call <vilib>:"NT Update Persistence.vi"("Persistence"=w515, "Name"=w517) -> ()  [unwired: 9 in, 1 out]
      }
    }
  }
  n324 = while {
    tunnel: w47 -> [w522]
    i -> [w525]
    stop <- FALSE stop-if-true
    n325 = Wait (ms)(milliseconds to wait=u32 100) -> ()  [unwired: 1 out]
    n326 = case shown="\"Playback\"" "Rec Mode" {
      tunnel: w525 -> [_ _ w540]
      tunnel: [u32 2829099 ("Base Color") u32 11141120 ("Target Color") w529] -> w521
      frame "Stop", Default {
        # "Reset the color, extra updates don't cost much"
      }
      frame "Record" {
      }
      frame "Playback" {
        # "Playback"
        n327 = Quotient & Remainder(x=w540, y=u32 50 ("milliseconds to wait")) -> (x-y*floor(x/y)=w536:u32)  [unwired: 1 out]
        n328 = Divide(x=w536, y=u32 50 ("milliseconds to wait")) -> (x/y=w533:dbl)
        n329 = Multiply(x=6.283185307179586, y=w533) -> (x*y=w538:dbl)
        n330 = Sine(x=w538) -> (sin(x)=w537:dbl)
        n331 = Absolute Value(x=w537) -> (abs(x)=w530:dbl)
        n332 = call "Interpolate RGB Color.vi"("Proportion"=w530, "Target Color"=u32 30976, "Base Color"=u32 2829099) -> ("Result Color"=w529:u32)  [unwired: 8 in]
      }
    }
    n333 = property class="Pane"(reference=w522, "PaneColor"=w521) -> ()  [unwired: 1 in, 2 out]
  }
  n334 = local write "Dashboard Tab"(T1."Drive" ("Dashboard Tab")) -> ()
  n335 = property on="On/Off" class="Bool (strict)"("Visible"=w15) -> ()  [unwired: 2 in, 2 out]
  n336 = property on="Motor" class="Clust (strict)"("Visible"=w15) -> ()  [unwired: 2 in, 2 out]
  n337 = property on="Progress" class="Clust (strict)"("Visible"=w15) -> ()  [unwired: 2 in, 2 out]
  n338 = property on="Test Ring" class="Ring (strict)"("Visible"=w15) -> ()  [unwired: 2 in, 2 out]
  n339 = property on="Rev/Fwd" class="Clust (strict)"("Visible"=w15) -> ()  [unwired: 2 in, 2 out]
  n340 = property on="Camera Settings" class="Clust (strict)"("Visible"=w15) -> ()  [unwired: 2 in, 2 out]
  n341 = while {
    tunnel: u16 1741 ("timeout ms (25000)") -> [w542]
    stop <- FALSE stop-if-true
    n342 = TCP Create Listener(10:w542) -> (0:w541:errorcluster, 3:w543:refnum<k5>)  [unwired: 4 in, 1 out]
    n343 = case shown="No Error" w541 {
      selector: w541 -> [w545 _]
      tunnel: w543 -> [w546 _]
      frame No Error {
        n344 = while {
          tunnel: w546 -> [w549]
          tunnel: w545 -> [w548]
          stop <- FALSE stop-if-true
          n345 = TCP Wait On Listener(8:w548, 11:w549) -> (0:w550:errorcluster, 4:w551:refnum<k5>)  [unwired: 2 in, 3 out]
          n346 = local write "TCP"(w551) -> ()
          n347 = case shown="No Error" w550 {
            frame No Error {
            }
            frame Error {
              n348 = Wait (ms)(milliseconds to wait=u32 1000) -> ()  [unwired: 1 out]
            }
          }
        }
      }
      frame Error {
        n349 = Wait (ms)(milliseconds to wait=u32 1000) -> ()  [unwired: 1 out]
      }
    }
  }
  n350 = local write "DB Camera Config"(w15) -> ()
  n351 = local write "Command Params"(string[][] [] ("Command Params")) -> ()
  n352 = global write "WPI_DashboardLogging Global.vi" "Recording"(w41) -> ()
  n353 = local write "Command Selection"(u16 0 ("milliseconds to wait")) -> ()
  n354 = local write "Rec Mode"(w41) -> ()
